vi "ALSO Filter Registration Types.vi"(9 "Valid Registration Types":T1[](array[typedef]), 10 "Requested Registration Types":T1[](array[typedef]), 11 "ControlEventHandler in":refnum<class "ControlEventHandler.lvclass">) -> (0 "error out":errorcluster, 3 "Array":T1[](array[typedef]))   [LabVIEW 2015]
uses:
  <vilib>/ErrorRing/Error Ring.xnode
  <vilib>/Utility/error.llb/Error Cluster From Error Code.vi
  EventHandler/ControlEventHandler/ControlEventHandler.lvclass
  <vilib>/event_ctls.llb/lveventtype.ctl
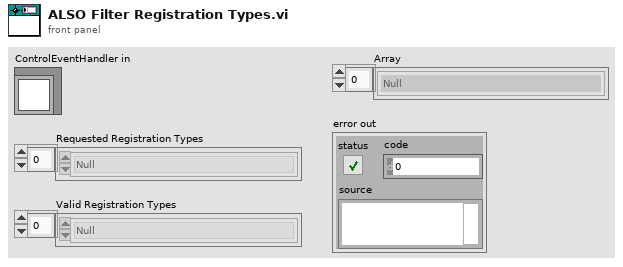
[diagram p1: front panel]
types:
  T1 = typedef "lveventtype.ctl" = enum32{"Null", "Timeout", "Annotation Menu Selection", "Annotation Menu Selection?", "App Instance Close", "App Instance Close?", "Autoscale Range Change", "Bookmark Info Change", "Cell Edit", "Cell Edit?", "Cursor Grab", "Cursor Grab?", "Cursor Menu Selection", "Cursor Menu Selection?", "Cursor Move", "Cursor Release", "Data Change", "Direction Change", "Display State Change", "Drag Ended", "Drag Enter", "Drag Leave", "Drag Over", "Drag Source Update", "Drag Starting", "Drag Starting?", "Drop", "Exec State Change", "Key Down", "Key Down?", "Key Repeat", "Key Repeat?", "Key Up", "Listbox Double Click", "Menu Activation?", "Menu Selection (App)", "Menu Selection? (App)", "Menu Selection (User)", "Mouse Down", "Mouse Down?", "Mouse Enter", "Mouse Leave", "Mouse Move", "Mouse Up", "Mouse Wheel", "NI Security User Change (App)", "Pane Size", "Panel Close", "Panel Close?", "Panel Resize", "Plot Attribute Change", "Scale Range Change", "Shortcut Menu Activation?", "Shortcut Menu Selection (App)", "Shortcut Menu Selection? (App)", "Shortcut Menu Selection (User)", "Tree Double Click", "Tree Drag", "Tree Drag?", "Tree Drop", "Tree Drop?", "Tree Item Close", "Tree Item Close?", "Tree Item Open", "Tree Item Open?", "User Event", "Value Change"}
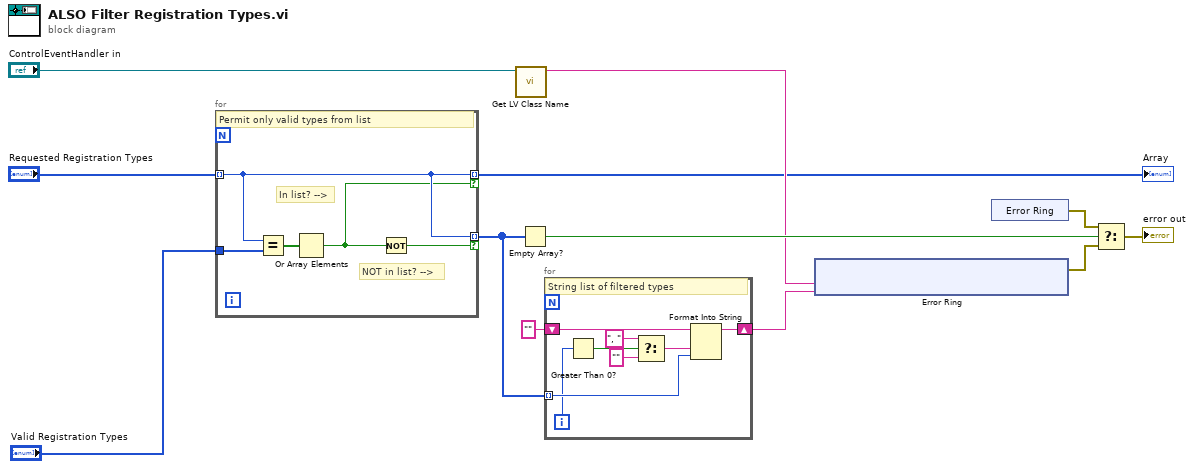
[diagram p0: block diagram]
diagram:
  n1 = for {
    tunnel: "Requested Registration Types" -> [w15] mode=indexing
    tunnel: "Valid Registration Types" -> [w17]
    tunnel: [w15] -> w5 mode=indexing if=w13
    tunnel: [w15] -> w10 mode=indexing if=w14
    # "NOT in list? -->"
    # "In list? -->"
    # "Permit only valid types from list"
    n2 = Equal?(x=w15, y=w17) -> (x = y?=w16:bool[])
    n3 = Or Array Elements(Boolean array=w16) -> (logical OR=w13:bool)
    n4 = Not(x=w13) -> (.not. x?=w14:bool)
  }
  "Array" <- w5
  n5 = call <vilib>:"Get LV Class Name.vi"("object"="ControlEventHandler in") -> ("class name"=w8:string)  [unwired: 9 in, 1 out]
  n6 = Empty Array?(array=w10) -> (empty?=w9:bool)
  n7 = for {
    tunnel: w10 -> [w23] mode=indexing
    shift-right: [w25] -> w12
    shift-left: "" -> [w24]
    i -> [w22]
    # "String list of filtered types"
    n8 = Greater Than 0?(x=w22) -> (x > 0?=w21:bool)
    n9 = Select(t=", ", s=w21, f="") -> (s? t:f=w18:string)
    n10 = Format Into String(initial string=w24, w18, w23) -> (resulting string=w25:string)  [unwired: 2 in, 1 out]
  }
  n11 = xnode "Error Ring"("parameter 0"=w8, "parameter 1"=w12) -> ("error out"=w4:errorcluster)
  n12 = xnode "Error Ring"() -> ("error out"=w3:errorcluster)
  n13 = Select(t=w3, s=w9, f=w4) -> (s? t:f=→"error out":errorcluster)
